vi "Export Built-ins.vi"(6 "Skip":cluster{"Functions":i32[], "Controls":i32[]}={"Functions"=[2371, 2060], "Controls"=[3503, 21820]}, 8 "error in (no error)":errorcluster, 9 "Scripting Ring (NaN)":refnum<vi>, 10 "LabVIEW Version Year (\"\"=This Version)":string, 11 "OutputDir (\"\"=..\\<AppDir>)":path) -> (0 "error out":errorcluster, 2 "Built-in Controls":cluster{"ControlsDir":path, "Control IDs":i32[]}, 3 "Built-in Functions":T1)   [LabVIEW 2018, in "Export-Built-ins.lvlib"]
uses:
  Export-Built-ins.lvlib
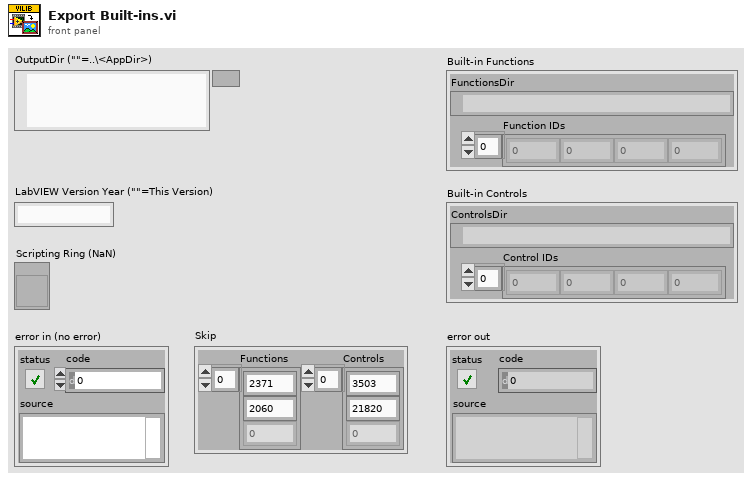
[diagram p1: front panel]
types:
  T1 = cluster{"FunctionsDir":path, "Function IDs":i32[]}
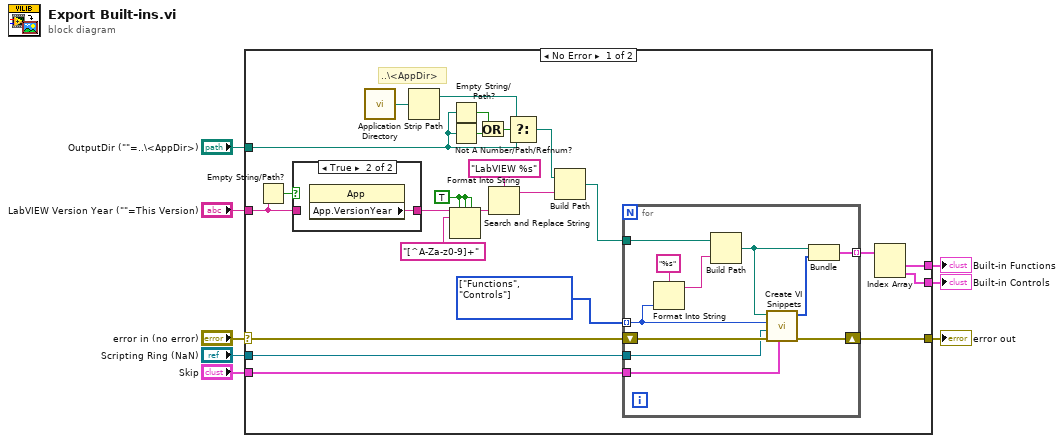
[diagram p0: block diagram]
diagram:
  n1 = case shown="No Error" "error in (no error)" {
    selector: "error in (no error)" -> [w32 w46]
    tunnel: "Scripting Ring (NaN)" -> [w23 _]
    tunnel: "LabVIEW Version Year (\"\"=This Version)" -> [w11 _]
    tunnel: [w21 _] -> w5
    tunnel: [w20 _] -> w4
    tunnel: "OutputDir (\"\"=..\\<AppDir>)" -> [w16 _]
    tunnel: [w13 w46] -> w2
    tunnel: "Skip" -> [w9 _]
    frame No Error {
      w27 = TRUE ("replace all? (F)")
      w30 = enum8{"Functions", "Controls"}[] [enum."Functions", enum."Controls"] items=["Functions", "Controls"] ("Type")
      # "..\\<AppDir>"
      n2 = Empty String/Path?(string/path=w11) -> (empty?=w10:bool)
      n3 = case shown="True" w10 {
        tunnel: [w33 w34] -> w12
        tunnel: w11 -> [w33 _]
        frame False {
        }
        frame True {
          n4 = property class="App"() -> ("App.VersionYear"=w34:string)  [unwired: 2 in, 2 out]
        }
      }
      n5 = call <vilib>:"Application Directory.vi"() -> ("Application Directory"=w31:path)
      n6 = Strip Path(path=w31) -> (stripped path=w15:path)  [unwired: 1 out]
      n7 = Search and Replace String(replace all?=w27, case sensitive?=w27, multiline?=w27, input string=w12, search string="[^A-Za-z0-9]+") -> (result string=w25:string)  [unwired: 3 in, 3 out]
      n8 = Empty String/Path?(string/path=w16) -> (empty?=w18:bool)
      n9 = Not A Number/Path/Refnum?(number/path/refnum=w16) -> (NaN/Path/Refnum?=w19:bool)
      n10 = Or(x=w18, y=w19) -> (x .or. y?=w17:bool)
      n11 = Format Into String(format string="LabVIEW %s", w25) -> (resulting string=w29:string)  [unwired: 2 in, 1 out]
      n12 = Select(t=w15, s=w17, f=w16) -> (s? t:f=w14:path)
      n13 = Build Path(base path=w14, name or relative path=w29) -> (appended path=w24:path)
      n14 = for {
        tunnel: w30 -> [w43] mode=indexing
        tunnel: w24 -> [w44]
        tunnel: [w39] -> w22 mode=indexing
        shift-right: [w38] -> w13
        shift-left: w32 -> [w45]
        tunnel: w23 -> [w37]
        tunnel: w9 -> [w35]
        n15 = Format Into String(format string="%s", w43) -> (resulting string=w42:string)  [unwired: 2 in, 1 out]
        n16 = Build Path(base path=w44, name or relative path=w42) -> (appended path=w36:path)
        n17 = call "Create VI Snippets.vi"("Skip"=w35, "error in (no error)"=w45, "Scripting Ring"=w37, "Type"=w43, "OutputDir"=w36) -> ("error out"=w38:errorcluster, "IDs"=w40:i32[])  [unwired: 5 in]
        n18 = Bundle("appended path"=w36, "IDs"=w40) -> (w39:cluster{"appended path":path, "IDs":i32[]})  [unwired: 1 in]
      }
      n19 = Index Array(array=w22) -> (element #1=w21:cluster{"appended path":path, "IDs":i32[]}, element #2=w20:cluster{"appended path":path, "IDs":i32[]})  [unwired: 2 in]
    }
    frame Error {
    }
  }
  "Built-in Functions" <- w5
  "Built-in Controls" <- w4
  "error out" <- w2
